vi "GetMetricById.vi"(10 "metric id":string, 11 "metrics in":T1[](array[typedef])) -> (1 "found":bool, 2 "metric":T1, 3 "metrics out":T1[](array[typedef]))   [LabVIEW 2017, in "DeviceModelHelpers.lvlib"]
uses:
  <vilib>/addons/InsightCM/Utilities/DeviceModelHelpers/DeviceModelHelpers.lvlib
  <vilib>/addons/InsightCM/MessageBus/Base/controls/Metric.ctl
  <vilib>/addons/InsightCM/MessageBus/Base/controls/KeyValuePair.ctl
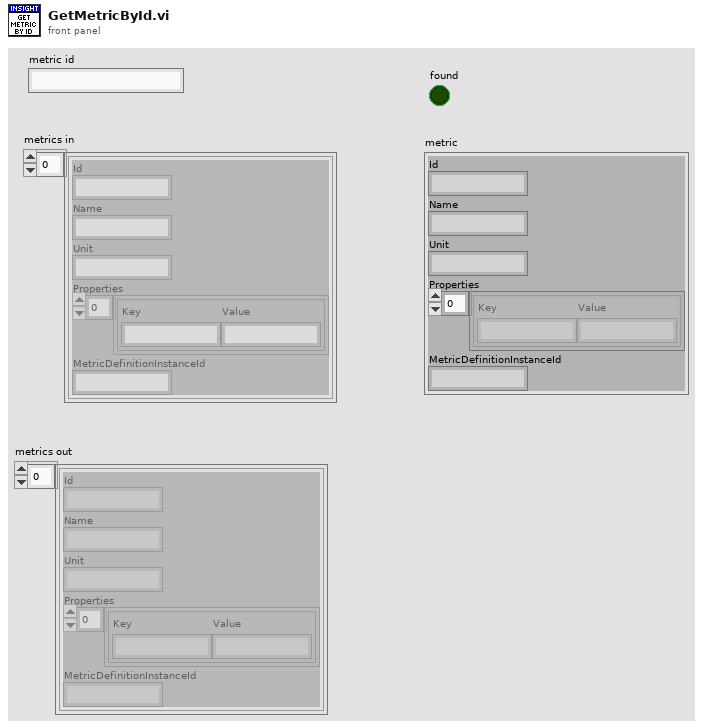
[diagram p1: front panel]
types:
  T1 = typedef "Metric.ctl" = cluster{"Id":string, "Name":string, "Unit":string, "Properties":T2[], "MetricDefinitionInstanceId":string}
  T2 = typedef "KeyValuePair.ctl" = cluster{"Key":string, "Value":string}
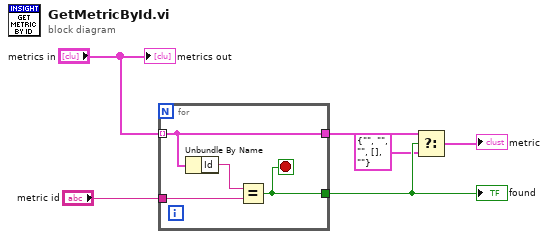
[diagram p0: block diagram]
diagram:
  n1 = for {
    tunnel: "metrics in" -> [w8] mode=indexing
    tunnel: "metric id" -> [w9]
    tunnel: [w8] -> w4
    tunnel: [w7] -> w5
    stop <- w7 stop-if-true
    n2 = Unbundle By Name(w8) -> ("Id"=w10:string)
    n3 = Equal?(x=w10, y=w9) -> (x = y?=w7:bool)
  }
  "found" <- w5
  n4 = Select(t=w4, s=w5, f=T1 {"Id"="", "Name"="", "Unit"="", "Properties"=[], "MetricDefinitionInstanceId"=""} ("MetricModel")) -> (s? t:f=→"metric":T1)
  "metrics out" <- "metrics in"
